vi "MDAQ_MsgCuller.vi"(10 "Main Cluster":T1 {"CV"."Temperature Array" scale=0.0..100.0}) -> (2 "Main Out":T1 {"CV"."Temperature Array" scale=0.0..100.0})   [LabVIEW 2021]
uses:
  GUI_Def.ctl
  Mode_Enum.ctl
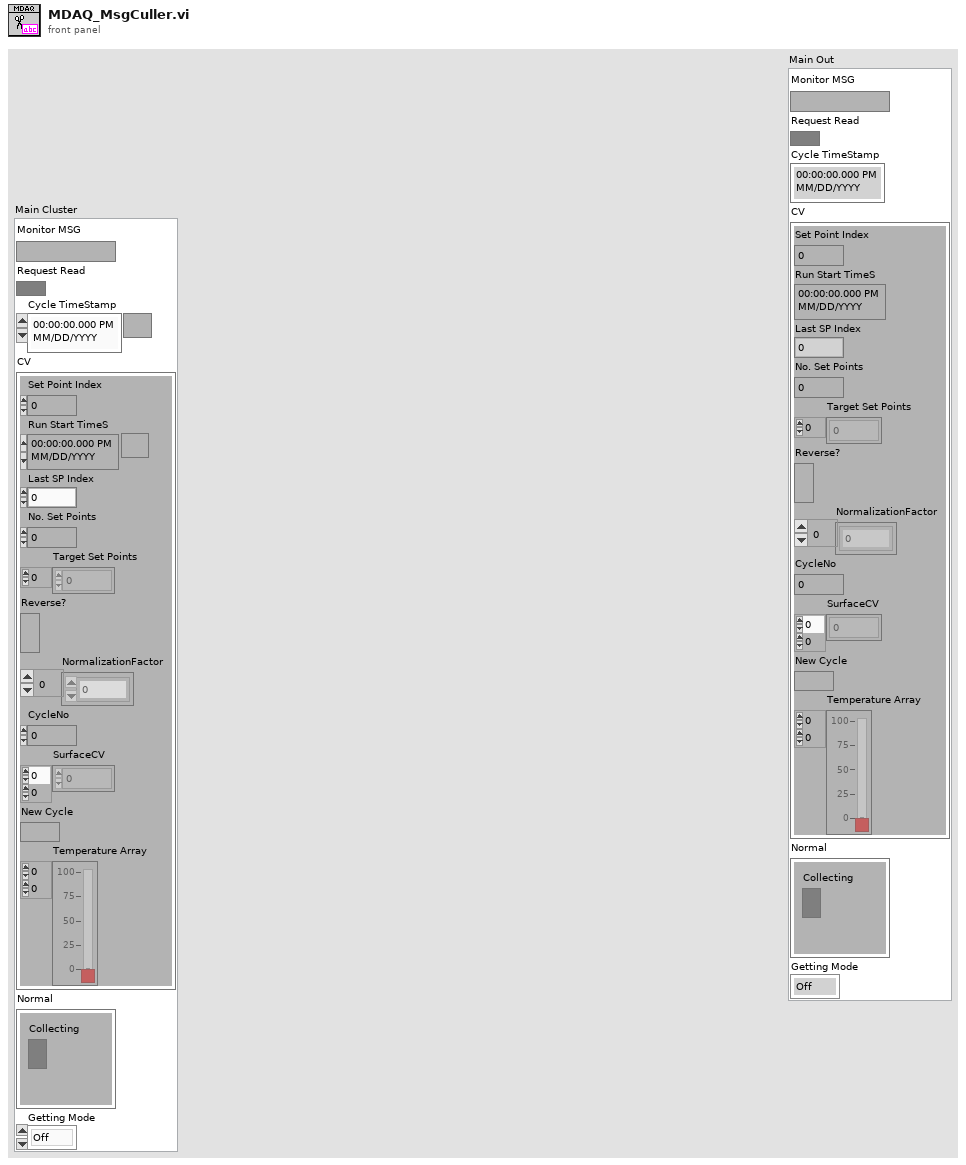
[diagram p1: front panel]
types:
  T1 = typedef "GUI_Def.ctl" = cluster{"Monitor MSG":string, "Request Read":bool, "Cycle TimeStamp":timestamp, "CV":cluster{"Set Point Index":u32, "Run Start TimeS":timestamp, "Last SP Index":u32, "No. Set Points":u32, "Target Set Points":i32[], "Reverse?":bool, "NormalizationFactor":i32[], "CycleNo":i32, "SurfaceCV":dbl[][], "New Cycle":bool, "Temperature Array":dbl[][]}, "Normal":cluster{"Collecting":bool}, "Getting Mode":T2}
  T2 = typedef "Mode_Enum.ctl" = enum16{"Off", "Normal", "CV+Temp", "CV"}
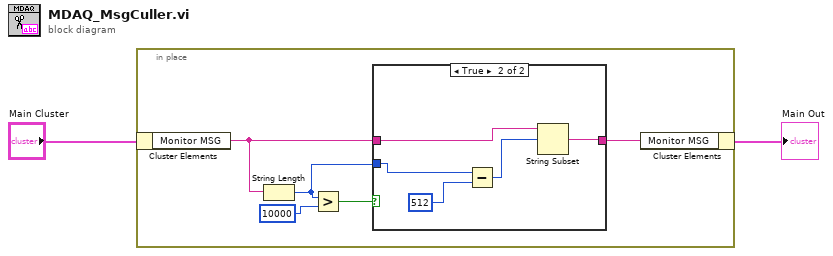
[diagram p0: block diagram]
diagram:
  n1 = in-place {
    n2 = in-place-cluster #1("Main Cluster") -> ("Monitor MSG"=w5:string)
    n3 = String Length(string=w5) -> (length=w3:i32)
    n4 = Greater?(x=w3, y=10000) -> (0:w6:bool)
    n5 = case shown="True" w6 {
      tunnel: w5 -> [w8 w12]
      tunnel: [w8 w13] -> w4
      tunnel: w3 -> [_ w11]
      frame False {
      }
      frame True {
        n6 = Subtract(x=w11, y=512) -> (x-y=w9:i32)
        n7 = String Subset(string=w12, offset (0)=w9) -> (substring=w13:string)  [unwired: 1 in]
      }
    }
    n8 = in-place-cluster #1("Monitor MSG"=w4) -> (→"Main Out":T1)
  }
